vi "SendMessage.vi"(5 "attributes":variant, 6 "timeout in ms (-1)":i32=-1, 7 "priority (-1, highest)":i32=-1, 8 "error in":errorcluster, 9 "data":variant, 10 "name":string, 11 "message ref in":refnum<class "CLM_PriorityLocalMessage.lvclass">) -> (0 "error out":errorcluster, 1 "priority used":i32, 3 "message ref out":refnum<class "CLM_PriorityLocalMessage.lvclass">, 4 "timed out?":bool)   [LabVIEW 2013, in "CLM_PriorityLocalMessage.lvclass"]
uses:
  CLM_PriorityLocalMessage.lvclass
  CLM_PriorityLocalMessage.lvclass/CLM_PriorityLocalMessage.ctl
  LocalMessage_Queue/CLM_LocalMessage_Queue.lvclass/CLM_LocalMessage_Queue.ctl
  LocalMessage_Queue/SendQueueMessage_Cluster.vi
  BufferIndexToPriority.vi
  PriorityToBufferIndex.vi
  LocalMessage/CLM_LocalMessage.lvclass
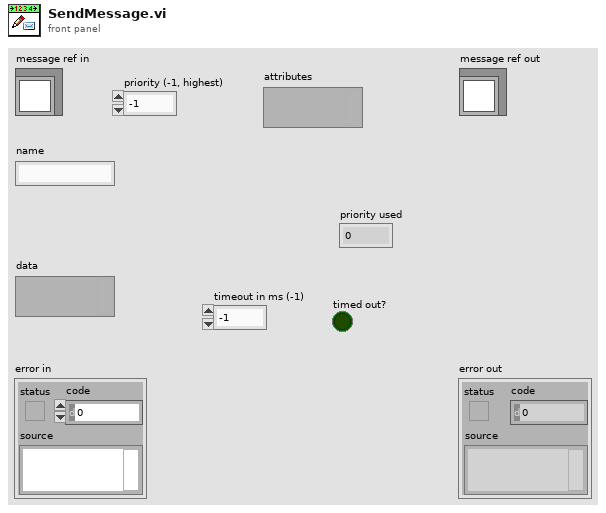
[diagram p1: front panel]
types:
  T1 = typedef "CLM_LocalMessage.lvclass/Message.ctl" = cluster{"name":string, "data":variant, "attributes":variant, "urgent":bool}
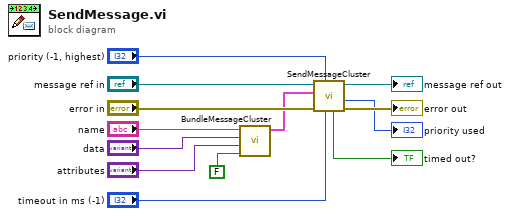
[diagram p0: block diagram]
diagram:
  n1 = call "BundleMessageCluster.vi"("urgent? (F)"=FALSE ("urgent"), "atributes"="attributes", "data"="data", "name"="name") -> ("message"=w1:T1)  [unwired: 7 in]
  n2 = call "SendMessageCluster.vi"("timeout in ms (-1)"="timeout in ms (-1)", "priority (-1, highest)"="priority (-1, highest)", "error in"="error in", "message"=w1, "queues in"="message ref in") -> ("error out"=→"error out":errorcluster, "priority used"=→"priority used":i32, "queues out"=→"message ref out":refnum<class "CLM_PriorityLocalMessage.lvclass">, "timed out?"=→"timed out?":bool)  [unwired: 3 in]
